vi "SetSettingsRequest.vi"(8 "error in (no error)":errorcluster, 10 "Data":variant, 11 "ModuleID":i32) -> (0 "error out":errorcluster)   [LabVIEW 2018, in "AcPwrModule.lvlib"]
uses:
  AcPwrModule.lvlib
  clEventType.ctl
  <vilib>/Utility/error.llb/Error Cluster From Error Code.vi
  <vilib>/ErrorRing/Error Ring.xnode
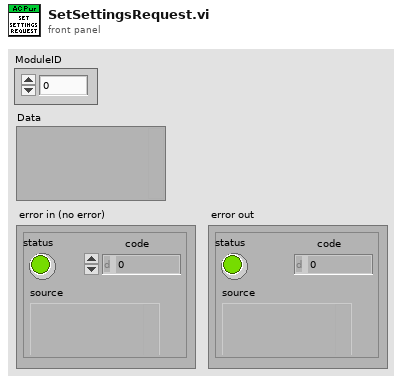
[diagram p1: front panel]
types:
  T1 = typedef "AcPwrModule.lvlib/clRequestEvents.ctl" = cluster{"StopRequest":refnum<user-event>, "PathToINI":refnum<user-event>, " LoadPlugin":refnum<user-event>, "ShowPanel":refnum<user-event>, "PrefDlg":refnum<user-event>, "InitAcPwr":refnum<user-event>, "Reset":refnum<user-event>, "Close":refnum<user-event>, "StopMeas":refnum<user-event>, "StartMeas":refnum<user-event>, "ConfigDevice":refnum<user-event>, "DeviceOn":refnum<user-event>, "DeviceOff":refnum<user-event>, "GetSettings":refnum<user-event>, "SetSettings":refnum<user-event>}
  T2 = typedef "AcPwrModule.lvlib/clEventType.ctl" = cluster{"ModuleID":i32, "Data":variant}
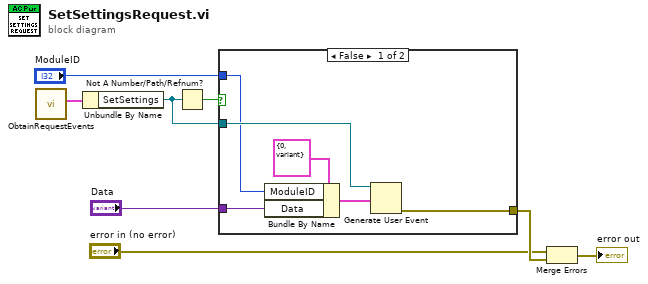
[diagram p0: block diagram]
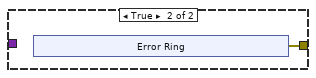
[diagram p2: hidden frame]
diagram:
  n1 = call "ObtainRequestEvents.vi"() -> ("clRequestEvents"=w5:T1)  [unwired: 10 in, 1 out]
  n2 = Unbundle By Name(w5) -> ("SetSettings"=w7:refnum<user-event>)
  n3 = Not A Number/Path/Refnum?(number/path/refnum=w7) -> (NaN/Path/Refnum?=w8:bool)
  n4 = case shown="False" w8 {
    tunnel: w7 -> [w13 _]
    tunnel: "ModuleID" -> [w11 _]
    tunnel: [w12 w15] -> w6
    tunnel: "Data" -> [w9 _]
    frame False {
      n5 = Bundle By Name(cluster=T2 {"ModuleID"=0, "Data"=variant} ("clEventType"), "ModuleID"=w11, "Data"=w9) -> (w14:T2)
      n6 = Generate User Event(user event=w13, event data cluster=w14) -> (error out=w12:errorcluster)  [unwired: 2 in, 1 out]
    }
    frame True {
      n7 = xnode "Error Ring"() -> ("error out"=w15:errorcluster)
    }
  }
  n8 = Merge Errors("error in (no error)", w6) -> (→"error out":errorcluster)
